vi "MakeHTMLList.vi"(3 "Escape Contents":bool, 4 "List Elements":string[](array[string]), 5 "List Type":enum16{"Ordered List", "Unordered List"}(ring)) -> (1 "List":string)   [LabVIEW 2019, in "ArgosLib.lvlib"]
uses:
  ArgosLib.lvlib
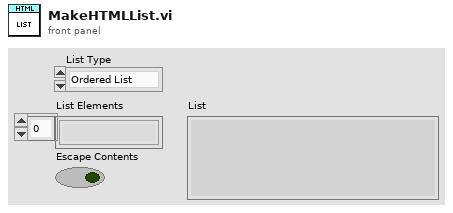
[diagram p1: front panel]
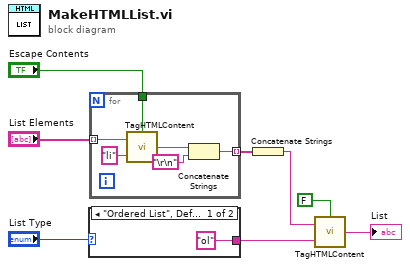
[diagram p0: block diagram]
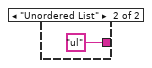
[diagram p2: hidden frame]
diagram:
  n1 = case shown="\"Ordered List\", Default" "List Type" {
    tunnel: ["ol" ("Tag") "ul" ("Tag")] -> w1
    frame "Ordered List", Default {
    }
    frame "Unordered List" {
    }
  }
  n2 = for {
    tunnel: "List Elements" -> [w16] mode=indexing
    tunnel: "Escape Contents" -> [w15]
    tunnel: [w12] -> w5 mode=indexing
    n3 = call "TagHTMLContent.vi"("Escape Contents"=w15, "Tag"="li", "Element Contents"=w16) -> ("Tagged Contents"=w13:string)
    n4 = Concatenate Strings(w13, "\r\n") -> (w12:string)
  }
  n5 = Concatenate Strings(w5) -> (w4:string)
  n6 = call "TagHTMLContent.vi"("Escape Contents"=FALSE, "Tag"=w1, "Element Contents"=w4) -> ("Tagged Contents"=→"List":string)
